vi "Lockout.vi"(0 "Locks":refnum<vi>, 1 "ID":i32, 2 "Queue System":refnum<vi>, 3 "Request Type":T1(ring), 4 "Request Array":i32[](array[numeric])=[0, 1, 2, 3, 4, 5, 6, 7, 8], 7 "Reactor Name":string, 8 "JSON Queue":refnum<vi>) -> (5 "Response":bool, 6 "Locks Held":i32[](array[numeric]))   [LabVIEW 2022 SP3]
doc: "If Request Type is Lock, returns true if the lock was successful\nIf Request Type is Release, returns true (and releases locks) only if all of the requested locks were owned by ID\nIf Request Type is Check, returns true only if the requested locks are held by ID\n\nIDs\n0 Open\n1-6 Chamber\n-1 System\n\nLock Indecies:\n0 Pump\n1 Shared Line 1\n2 Shared Line 2\n3-8 Chamber Sets 1-6"
uses:
  <vilib>/Utility/error.llb/whitespace.ctl
  <vilib>/Utility/error.llb/Trim Whitespace One-Sided.vi
panel:
  out "Value":i32[](array[numeric])
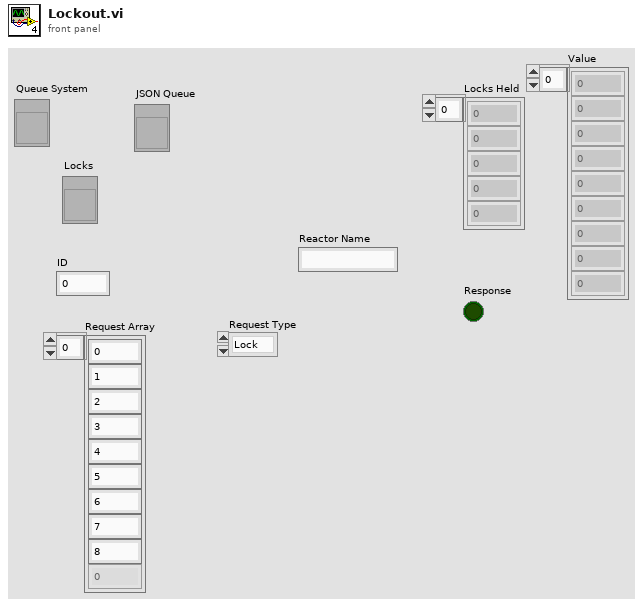
[diagram p1: front panel]
types:
  T1 = enum16{"Lock", "Release", "Check", "Check All", "Release All"}
  T2 = typedef "whitespace.ctl" = u16
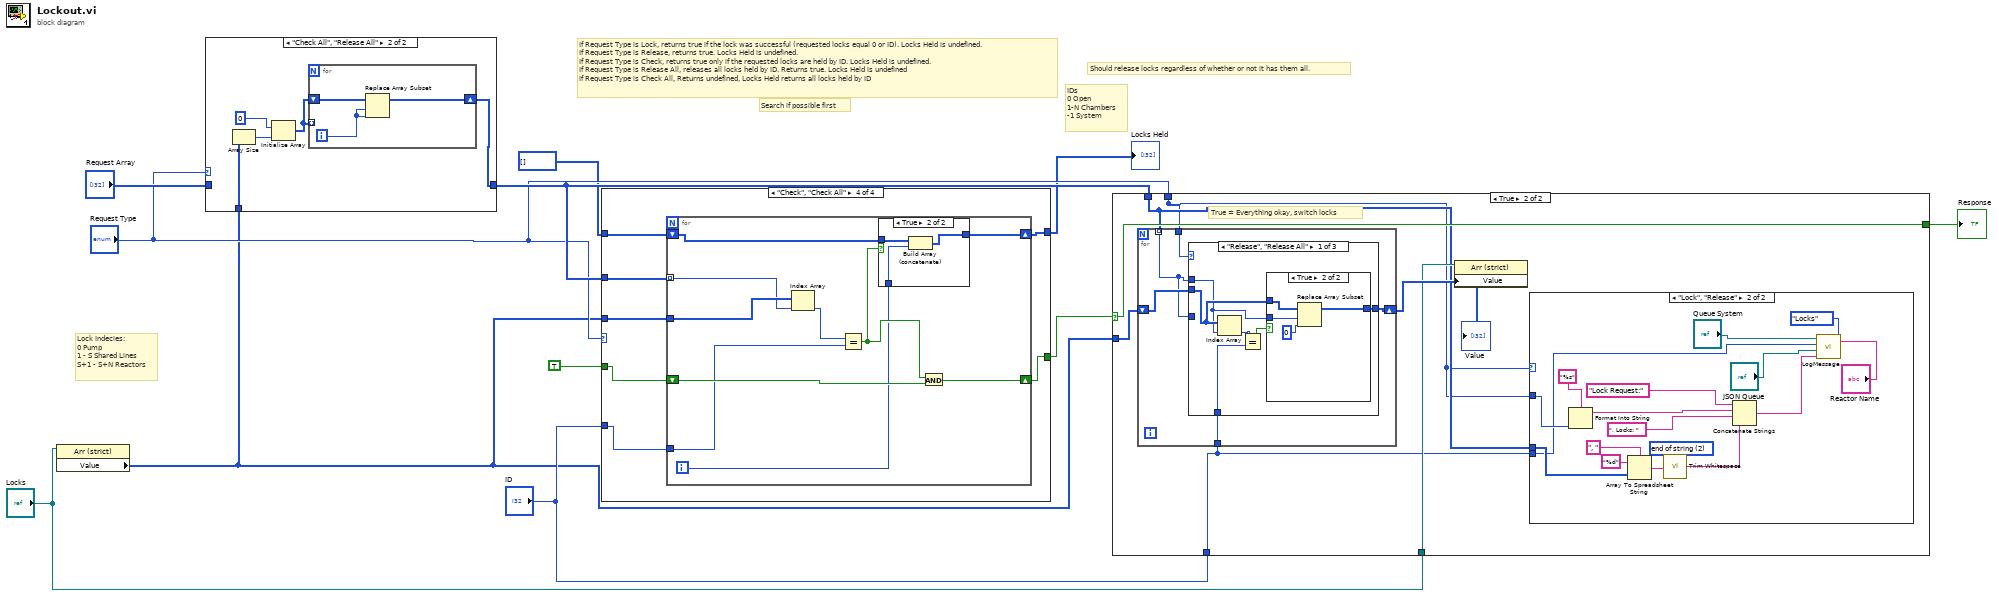
[diagram p0: block diagram]
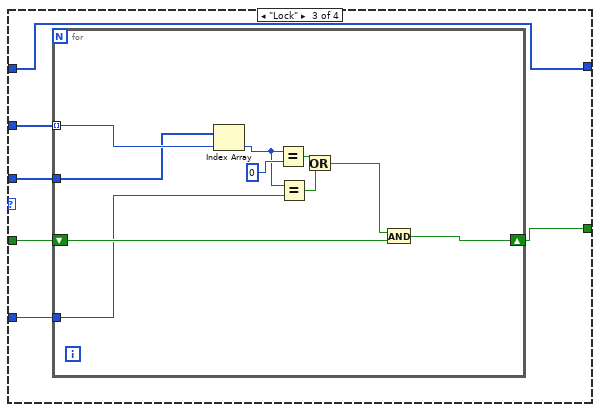
[diagram p5: hidden frame]
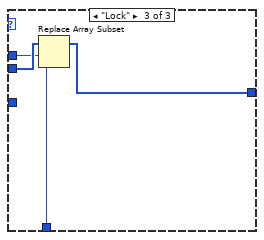
[diagram p11: hidden frame]
diagram:
  # "Should release locks regardless of whether or not it has them all."
  # "Lock Indecies:\n0 Pump\n1 - S Shared Lines\nS+1 - S+N Reactors"
  # "Search if possible first"
  # "IDs\n0 Open\n1-N Chambers\n-1 System"
  # "If Request Type is Lock, returns true if the lock was successful (requested locks equal 0 or ID). Locks Held is undefined.\nIf Request Type is Release, returns true. Locks Held is undefined.\nIf Request Type is Check, returns true only if the requested locks are held by ID. Locks Held is undefined.\nIf Request Type is Release All, releases all locks held by ID. Returns true. Locks Held is undefined\nIf Request Type is Check All, Returns undefined, Locks Held returns all locks held by ID"
  n1 = property class="Arr (strict)"(reference="Locks") -> ("Value"=w1:i32[])  [unwired: 1 in, 2 out]
  n2 = case shown="\"Check All\", \"Release All\"" "Request Type" {
    tunnel: [w12 w13] -> w7
    tunnel: "Request Array" -> [w12 _]
    tunnel: w1 -> [_ w16]
    frame Default {
    }
    frame "Check All", "Release All" {
      n3 = Array Size(array=w16) -> (size(s)=w17:i32)
      n4 = Initialize Array(0, w17) -> (w14:i32[])
      n5 = for {
        tunnel: w14 -> [_] mode=indexing
        shift-right: [w18] -> w13
        shift-left: w14 -> [w20]
        i -> [w19]
        n6 = Replace Array Subset(array=w20, new element=w19, index=w19) -> (w18:i32[])
      }
    }
  }
  n7 = case shown="\"Check\", \"Check All\"" "Request Type" {
    tunnel: TRUE -> [w22 w24 w30 w45]
    tunnel: [w22 w24 w29 w47] -> w10
    tunnel: w1 -> [_ _ w28 w42]
    tunnel: "ID" -> [_ _ w27 w46]
    tunnel: w7 -> [_ _ w26 w41]
    tunnel: i32[] [] -> [w21 w23 w25 w44]
    tunnel: [w21 w23 w25 w43] -> w3
    frame Default {
    }
    frame "Release All" {
    }
    frame "Lock" {
      n8 = for {
        tunnel: w26 -> [w40] mode=indexing
        tunnel: w28 -> [w39]
        shift-right: [w37] -> w29
        shift-left: w30 -> [w38]
        tunnel: w27 -> [w36]
        n9 = Index Array(array=w39, index=w40) -> (element=w33:i32)
        n10 = Equal?(x=w33, y=0) -> (x = y?=w34:bool)
        n11 = Equal?(x=w33, y=w36) -> (x = y?=w32:bool)
        n12 = Or(x=w34, y=w32) -> (x .or. y?=w31:bool)
        n13 = And(x=w31, y=w38) -> (x .and. y?=w37:bool)
      }
    }
    frame "Check", "Check All" {
      n14 = for {
        tunnel: w42 -> [w57]
        shift-right: [w55] -> w47
        shift-left: w45 -> [w56]
        tunnel: w46 -> [w54]
        shift-right: [w50] -> w43
        shift-left: w44 -> [w51]
        tunnel: w41 -> [w48] mode=indexing
        i -> [w49]
        n15 = Index Array(array=w57, index=w48) -> (element=w53:i32)
        n16 = Equal?(x=w53, y=w54) -> (x = y?=w52:bool)
        n17 = case shown="True" w52 {
          tunnel: w51 -> [w58 w61]
          tunnel: w49 -> [_ w60]
          tunnel: [w58 w59] -> w50
          frame False {
          }
          frame True {
            n18 = Build Array (concatenate)(w61, w60) -> (w59:i32[])
          }
        }
        n19 = And(x=w52, y=w56) -> (x .and. y?=w55:bool)
      }
    }
  }
  "Locks Held" <- w3
  n20 = case shown="True" w10 {
    selector: w10 -> [w62 w69]
    tunnel: w7 -> [_ w64]
    tunnel: w1 -> [_ w68]
    tunnel: "ID" -> [_ w65]
    tunnel: "Request Type" -> [_ w63]
    tunnel: [w62 w69] -> w2
    tunnel: "Locks" -> [_ w66]
    frame False {
    }
    frame True {
      # "True = Everything okay, switch locks"
      n21 = for {
        tunnel: w64 -> [w87] mode=indexing
        tunnel: w65 -> [w91]
        tunnel: w63 -> [w90]
        shift-right: [w88] -> w67
        shift-left: w68 -> [w89]
        n22 = case shown="\"Release\", \"Release All\"" w90 {
          tunnel: w89 -> [w94 w103 w107]
          tunnel: w87 -> [w93 _ w106]
          tunnel: w91 -> [w96 _ w105]
          tunnel: [w92 w103 w104] -> w88
          tunnel: w87 -> [_ _ _]
          frame "Release", "Release All" {
            n23 = Index Array(array=w94, index=w93) -> (element=w97:i32)
            n24 = Equal?(x=w97, y=w96) -> (x = y?=w95:bool)
            n25 = case shown="True" w95 {
              tunnel: w94 -> [w98 w102]
              tunnel: w93 -> [_ w101]
              tunnel: [w98 w99] -> w92
              frame False {
              }
              frame True {
                n26 = Replace Array Subset(array=w102, new element=0 ("new element/subarray"), index=w101) -> (w99:i32[])
              }
            }
          }
          frame "Check", "Check All" {
          }
          frame "Lock" {
            n27 = Replace Array Subset(array=w107, new element=w105, index=w106) -> (w104:i32[])
          }
        }
      }
      "Value" <- w67
      n28 = property class="Arr (strict)"(reference=w66, "Value"=w67) -> ()  [unwired: 1 in, 2 out]
      n29 = case shown="\"Lock\", \"Release\"" w63 {
        tunnel: w65 -> [_ w73]
        tunnel: w63 -> [_ w85]
        tunnel: w64 -> [_ w80]
        frame "Check", Default {
        }
        frame "Lock", "Release" {
          w78 = T2 2 items=["both", "start of string", "end of string"] ("location (both)")
          n30 = Format Into String(format string="%s", w85) -> (resulting string=w83:string)  [unwired: 2 in, 1 out]
          n31 = Array To Spreadsheet String(delimiter (Tab)=", ", array=w80, 3:"%d" ("format string")) -> (spreadsheet string=w79:string)
          n32 = call <vilib>:"Trim Whitespace.vi"("string"=w79, "location (both)"=w78) -> ("trimmed string"=w77:string)
          n33 = Concatenate Strings("Lock Request:" ("Log Entry"), w83, ", Locks: " ("string"), w77) -> (w75:string)
          n34 = call "LogMessage.vi"("Type"=enum16{"Locks", "Warning"}."Locks", "Reactor Name"="Reactor Name", "Log Entry"=w75, "System JSON Queue"="JSON Queue", "ID Number"=w73, "System Queue"="Queue System") -> ()
        }
      }
    }
  }
  "Response" <- w2
